vi "receivePressureData.vi"(8 "error in (no error)":errorcluster, 11 "ILC in":refnum<class "ILC.lvclass">) -> (0 "error out":errorcluster, 3 "ILC out":refnum<class "ILC.lvclass">)   [LabVIEW 2015, in "ILCCommon.lvlib" / "ILC.lvclass"]
uses:
  <userlib>/Common/ILC/ILC/ILC.lvclass
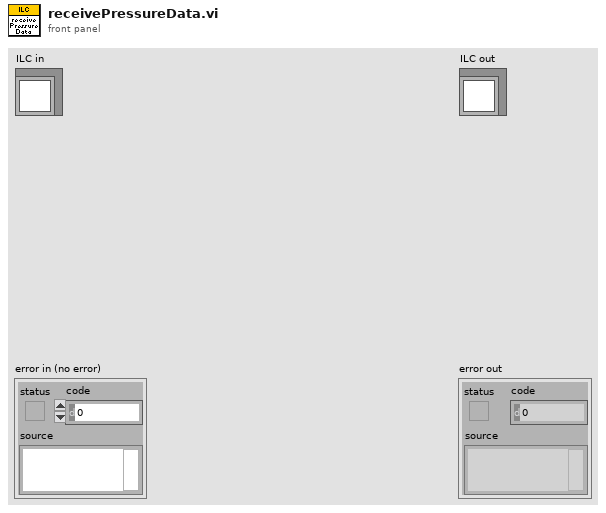
[diagram p1: front panel]
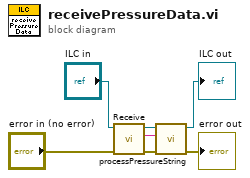
[diagram p0: block diagram]
diagram:
  n1 = call-dynamic "Receive.vi"("error in (no error)"="error in (no error)", "ILC in"="ILC in") -> ("error out"=w6:errorcluster, "Response"=w3:string, "ILC out"=w5:refnum<class "ILC.lvclass">)  [unwired: 7 in]
  n2 = call <userlib>:"processPressureString.vi"("error in (no error)"=w6, "stringRead"=w3, "ILC in"=w5) -> ("error out"=→"error out":errorcluster, "ILC out"=→"ILC out":refnum<class "ILC.lvclass">)  [unwired: 7 in]
